vi "Main Process Outgoing Messages.vi"(8 "error in (no error)":errorcluster, 11 "J1939 Main Configuration":T1={"Parameters"={"J1939 XNET Settings"={"XNET Database"="", "XNET Cluster"="", "CAN Port"="", "Baud rate [Bd]"=0, "Termination"=0, "Incoming Rate"=0, "Outcoming Rate"=1, "Write Decimation"=1}, "Incoming Single Point Configuraiton"={"Incoming Single Point Frame"={"ID"=[], "Conversion"=[], "Channel Array Positions"=[], "Frame Length"=[]}, "Channel Pairs"={"Chan Refs"=[], "Previous Chan Values"=[]}, "Read FIFO"=refnum}, "Outgoing Cyclic Configuraiton"={"Outgoing Cyclic Frame"={"ID"=[], "Conversion"=[], "Channel Array Positions"=[], "Frame Length"=[], "Transmit Propreties"=[]}, "Channel Pairs"={"Block Data Refs"=[], "Previous Chan Values"=[]}, "Write FIFO"=refnum}, "J1939 Monitor Settings"={"J1939 Network Address"=0, "Name"=0}, "Simulated Addresses"=[], "Simulated Addresses LUT"=variant, "Name"=""}, "Name"="", "J1939 Cluster"={"Processed Incoming"=refnum, "Current Device Address"=0, "Processed Outgoing"=refnum, "Process Outgoing"=refnum, "Name"=0}, "References"={"BAM Buffer"=refnum, "CM Buffer"=refnum, "CM Gen"=refnum, "BAM Gen"=refnum, "Address Claims"=refnum, "RQST"=refnum}, "Frame In"="", "Frame Out"="", "Incoming Timeout"=0, "Outgoing Timeout"=0, "Listener ID"=refnum, "Process"=refnum, "Data Ref"=refnum, "Scale Ref"=refnum, "Incoming Direct Access"={"Offset"=0, "Length"=0}, "Outgoing Direct Access"={"Offset"=0, "Length"=0}, "TCP Mngr Ref"=refnum, "Name and Address"="", "Simulated Addresses"=[], "Simulated Addresses LUT"=variant} {"Simulated Addresses"."Simulated Addresses"."J1939 XNET Settings"."Name" format="%.0x"; "Simulated Addresses"."Simulated Addresses"."DM1 Data"."Data Reference" format="%.0x"; "Simulated Addresses"."Simulated Addresses"."DM1 Enable?"."Data Reference" format="%.0x"; "Simulated Addresses"."Simulated Addresses"."DM2 Data"."Data Reference" format="%.0x"; "Simulated Addresses"."Simulated Addresses"."DM2 Enable?"."Data Reference" format="%.0x"; "Parameters"."Simulated Addresses"."Simulated Addresses"."J1939 XNET Settings"."Name" format="%.0x"; "Parameters"."J1939 Monitor Settings"."Name" format="%.0x"; "Parameters"."Outgoing Cyclic Configuraiton"."Channel Pairs"."Block Data Refs"."Data Reference" format="%.0x"; "Parameters"."Outgoing Cyclic Configuraiton"."Outgoing Cyclic Frame"."Transmit Propreties"."Transmit Time" format="%#_p"; "Parameters"."J1939 XNET Settings"."Termination" items=["Off", "On"]; "Parameters"."Incoming Single Point Configuraiton"."Channel Pairs"."Chan Refs" format="%.0x"}) -> (0 "error out":errorcluster)   [LabVIEW 2015, in "J1939 Addon Engine.lvlib"]
uses:
  J1939 Addon Engine.lvlib
  Types/Configuration Cluster.ctl
  <vilib>/NI/NI VeriStand Inline Async API/_VS Inline Async API/Process/Process.lvclass
  Types/Process Parameters.ctl
  Shared/Types/XNET Settings.ctl
  Types/Incoming Single Point Configuration.ctl
  Types/Incoming Single Point Frame Pairs.ctl
  Shared/Types/Incoming Single Point Channel Pairs.ctl
  <vilib>/NI Veristand/Custom Device API/Data Reference.ctl
  Types/Outgoing Cyclic Configuration.ctl
  Types/Outgoing Cyclic Frame Pairs.ctl
  Shared/Types/XNET Frame Event Properties.ctl
  Shared/Types/Outgoing Cyclic Channel Pairs.ctl
  <vilib>/NI Veristand/Custom Device API/Block Data Reference.ctl
  Shared/Types/Monitor Settings.ctl
  Types/Simulated Settings.ctl
  Shared/Types/Compiled Simulated Settings.ctl
  Types/DTC FIFOs.ctl
  Shared/J1939 Multi Packet Frame/Types/Setup Information Cluster.ctl
  <vilib>/xnet/xnet.llb/XNET Frame CAN.ctl
  <vilib>/xnet/xnet.llb/XNET Frame Type CAN.ctl
  Shared/J1939 Utilities/Types/CAN Outgoing Message Cluster.ctl
  Shared/J1939 Multi Packet Frame/Types/TP List References.ctl
  Shared/J1939 Multi Packet Frame/Types/BAM Buffer Connections List_Ref.ctl
  Shared/J1939 Multi Packet Frame/Types/TP Buffer Connection Cluster.ctl
  Shared/J1939 Multi Packet Frame/Types/Connection Mode Generation Connection Ref.ctl
  Shared/J1939 Multi Packet Frame/Types/Connection Mode Generation Connection Cluster.ctl
  Shared/J1939 Multi Packet Frame/Types/BAM Generation Connections List_Ref.ctl
  Shared/J1939 Multi Packet Frame/Types/BAM Generation Connection Cluster.ctl
  Shared/J1939 Multi Packet Frame/Types/Address Table Reference.ctl
  Shared/J1939 Multi Packet Frame/Types/RQST Lookup Table Reference.ctl
  Types/Data Lookup Table Reference.ctl
  Types/Datatable Lookup DVR.ctl
  Types/Conversion Lookup Table Reference.ctl
  Shared/J1939 Multi Packet Frame/Types/RQST Comm Lookup Table_Ref.ctl
  Shared/STM/Connection Manager/stm_ManagerStateVariables.ctl
  Shared/STM/TCP/stm_TCP Connection Info.ctl
  Shared/STM/_SubVIs/stm_MetaDataElement.ctl
  Shared/STM/Connection Manager/stm_TCPConnectionProperties.ctl
  Shared/J1939 Multi Packet Frame/J1939 Periodic Messages/SubVIs/Periodic Message Generator Cluster.ctl
  <vilib>/NI/NI VeriStand Inline Async API/_VS Inline Async API/Process/Process.lvclass/Process.ctl
  Shared/J1939 Multi Packet Frame/SubVIs/Read Queued Outgoing Messages.vi
  Shared/J1939 Multi Packet Frame/SubVIs/Process Outgoing Messages by Frame Type.vi
  Shared/J1939 Multi Packet Frame/J1939 Periodic Messages/Periodic Message Generator.vi
  Shared/J1939 Multi Packet Frame/SubVIs/Connection Mode Generation Queue Messages.vi
  <vilib>/NI/NI VeriStand Inline Async API/_VS Inline Async API/Error Handling Process/SubVIs/Error.ConvertArray.vi
  Shared/J1939 Utilities/Check Output Message Frame Type.vi
  Shared/J1939 Multi Packet Frame/J1939 Multi Packet Frames/BAM Generation.vi
  Shared/J1939 Multi Packet Frame/SubVIs/BAM Generation Connections List_Actions.vi
  Shared/J1939 Multi Packet Frame/SubVIs/BAM Generation Create New TP Connection.vi
  Shared/J1939 Multi Packet Frame/J1939 Multi Packet Frames/Connection Mode Generation.vi
  Shared/J1939 Multi Packet Frame/SubVIs/Connection Mode Generation Connections List_Actions.vi
  Shared/J1939 Multi Packet Frame/SubVIs/Connection Mode Generation Search for Connection (Local Message).vi
  Shared/J1939 Multi Packet Frame/SubVIs/Connection Mode Generation Create New TP Connection.vi
  Convert Signals to Frame by ID.vi
  Shared/J1939 Multi Packet Frame/SubVIs/Connection Mode Generation Get Next Messages.vi
  Shared/J1939 Utilities/SubVIs/TP.Conn Abort.vi
  Shared/J1939 Utilities/Common Conversions.vi
  Shared/J1939 Utilities/SubVIs/Convert CAN Arb ID to J1939 ID.vi
  Shared/J1939 Utilities/Common Messages.vi
  Shared/J1939 Utilities/SubVIs/TP.CM BAM.vi
  Shared/J1939 Utilities/SubVIs/TP.DT.vi
  Shared/J1939 Utilities/SubVIs/TP.CM RTS.vi
  Conversion Lookup Table Get Conversion Parameter.vi
  Data Lookup Table Get Signals (Range).vi
  Shared/J1939 Utilities/SubVIs/Convert J1939 ID to CAN Arb ID.vi
  Shared/J1939 Multi Packet Frame/SubVIs/Connection Mode Generation Connections List.vi
  Shared/J1939 Multi Packet Frame/SubVIs/BAM Generation Queue Messages.vi
  Shared/J1939 Multi Packet Frame/SubVIs/BAM Generation Connections List.vi
  Shared/J1939 Multi Packet Frame/SubVIs/BAM Generation Search for Connection (Local Message).vi
  <vilib>/xnet/xnet.llb/XNET Convert.vi
  <vilib>/xnet/xnet.llb/XNET Convert (Signal to Frame Raw).vi
  Data Lookup Table.vi
  Conversion Lookup Table.vi
  Shared/J1939 Utilities/J1939 Utilities.lvlib
  <vilib>/NI VeriStand/Custom Device API/Custom Device API.lvlib
  Shared/J1939 Addon Shared.lvlib
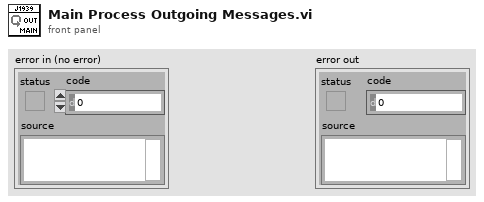
[diagram p1: front panel]
types:
  T1 = typedef "J1939 Addon Engine.lvlib/Configuration Cluster.ctl" = cluster{"Parameters":T2, "Name":string, "J1939 Cluster":T17, "References":T18, "Frame In":refnum<k21>, "Frame Out":refnum<k21>, "Incoming Timeout":u32, "Outgoing Timeout":u32, "Listener ID":refnum<k5>, "Process":refnum<class "Process.lvclass">, "Data Ref":T24, "Scale Ref":T25, "Incoming Direct Access":cluster{"Offset":u32, "Length":u32}, "Outgoing Direct Access":cluster{"Offset":u32, "Length":u32}, "TCP Mngr Ref":T26, "Name and Address":string, "Simulated Addresses":T14[], "Simulated Addresses LUT":variant}
  T2 = typedef "J1939 Addon Engine.lvlib/Process Parameters.ctl" = cluster{"J1939 XNET Settings":T3, "Incoming Single Point Configuraiton":T4, "Outgoing Cyclic Configuraiton":T8, "J1939 Monitor Settings":T13, "Simulated Addresses":T14[], "Simulated Addresses LUT":variant, "Name":string}
  T3 = typedef "J1939 Addon Shared.lvlib/XNET Settings.ctl" = cluster{"XNET Database":refnum<k21>, "XNET Cluster":refnum<k21>, "CAN Port":string, "Baud rate [Bd]":u32, "Termination":u32, "Incoming Rate":u32, "Outcoming Rate":u32, "Write Decimation":u32}
  T4 = typedef "J1939 Addon Engine.lvlib/Incoming Single Point Configuration.ctl" = cluster{"Incoming Single Point Frame":T5, "Channel Pairs":T6, "Read FIFO":refnum<k33>}
  T5 = typedef "J1939 Addon Engine.lvlib/Incoming Single Point Frame Pairs.ctl" = cluster{"ID":u32[], "Conversion":refnum<k21>[], "Channel Array Positions":cluster{"Offset":u32, "Length":u32}[], "Frame Length":u32[]}
  T6 = typedef "J1939 Addon Shared.lvlib/Incoming Single Point Channel Pairs.ctl" = cluster{"Chan Refs":T7[], "Previous Chan Values":dbl[]}
  T7 = typedef "Custom Device API.lvlib/Data Reference.ctl" = i32
  T8 = typedef "J1939 Addon Engine.lvlib/Outgoing Cyclic Configuration.ctl" = cluster{"Outgoing Cyclic Frame":T9, "Channel Pairs":T11, "Write FIFO":refnum<k33>}
  T9 = typedef "J1939 Addon Engine.lvlib/Outgoing Cyclic Frame Pairs.ctl" = cluster{"ID":u32[], "Conversion":refnum<k21>[], "Channel Array Positions":cluster{"Offset":u32, "Length":u32}[], "Frame Length":u32[], "Transmit Propreties":T10[]}
  T10 = typedef "J1939 Addon Shared.lvlib/XNET Frame Event Properties.ctl" = cluster{"Transmit trigger":enum16{"Channel value change"}, "Enable software cyclic trigger":bool, "Transmit Time":dbl}
  T11 = typedef "J1939 Addon Shared.lvlib/Outgoing Cyclic Channel Pairs.ctl" = cluster{"Block Data Refs":T12[], "Previous Chan Values":dbl[]}
  T12 = typedef "Custom Device API.lvlib/Block Data Reference.ctl" = cluster{"Data Reference":T7, "Offset":u64, "Length":u64}
  T13 = typedef "J1939 Addon Shared.lvlib/Monitor Settings.ctl" = cluster{"J1939 Network Address":u8, "Name":u64}
  T14 = typedef "J1939 Addon Engine.lvlib/Simulated Settings.ctl" = cluster{"Simulated Addresses":T15, "FIFOs":T16}
  T15 = typedef "J1939 Addon Shared.lvlib/Compiled Simulated Settings.ctl" = cluster{"J1939 XNET Settings":T13, "DM1 Data":T12[], "DM1 Data":dbl[], "DM1 Enable?":T12[], "DM1 Enable?":dbl[], "DM2 Data":T12[], "DM2 Data":dbl[], "DM2 Enable?":T12[], "DM2 Enable?":dbl[]}
  T16 = typedef "J1939 Addon Engine.lvlib/DTC FIFOs.ctl" = cluster{"DM1 Data":refnum<k33>, "DM1 Enable?":refnum<k33>, "DM2 Data":refnum<k33>, "DM2 Enable?":refnum<k33>, "DM1 Reset?":refnum<k33>, "DM2 Reset?":refnum<k33>}
  T17 = typedef "J1939 Addon Engine.lvlib/Setup Information Cluster.ctl" = cluster{"Processed Incoming":refnum<queue>, "Current Device Address":u8, "Processed Outgoing":refnum<queue>, "Process Outgoing":refnum<queue>, "Name":u64}
  T18 = typedef "J1939 Addon Engine.lvlib/TP List References.ctl" = cluster{"BAM Buffer":T19, "CM Buffer":T19, "CM Gen":T20, "BAM Gen":T21, "Address Claims":T22, "RQST":T23}
  T19 = typedef "J1939 Addon Engine.lvlib/BAM Buffer Connections List_Ref.ctl" = refnum<data-value>
  T20 = typedef "J1939 Addon Engine.lvlib/Connection Mode Generation Connection Ref.ctl" = refnum<data-value>
  T21 = typedef "J1939 Addon Engine.lvlib/BAM Generation Connections List_Ref.ctl" = refnum<data-value>
  T22 = typedef "J1939 Addon Engine.lvlib/Address Table Reference.ctl" = refnum<data-value>
  T23 = typedef "J1939 Addon Engine.lvlib/RQST Lookup Table Reference.ctl" = refnum<data-value>
  T24 = typedef "J1939 Addon Engine.lvlib/Data Lookup Table Reference.ctl" = refnum<data-value>
  T25 = typedef "J1939 Addon Engine.lvlib/Conversion Lookup Table Reference.ctl" = refnum<data-value>
  T26 = typedef "J1939 Addon Shared.lvlib/RQST Comm Lookup Table_Ref.ctl" = refnum<data-value>
  T27 = typedef "J1939 Addon Engine.lvlib/Periodic Message Generator Cluster.ctl" = cluster{"Arb ID":u32, "Timeout":u32, "Start Timeout":u32}
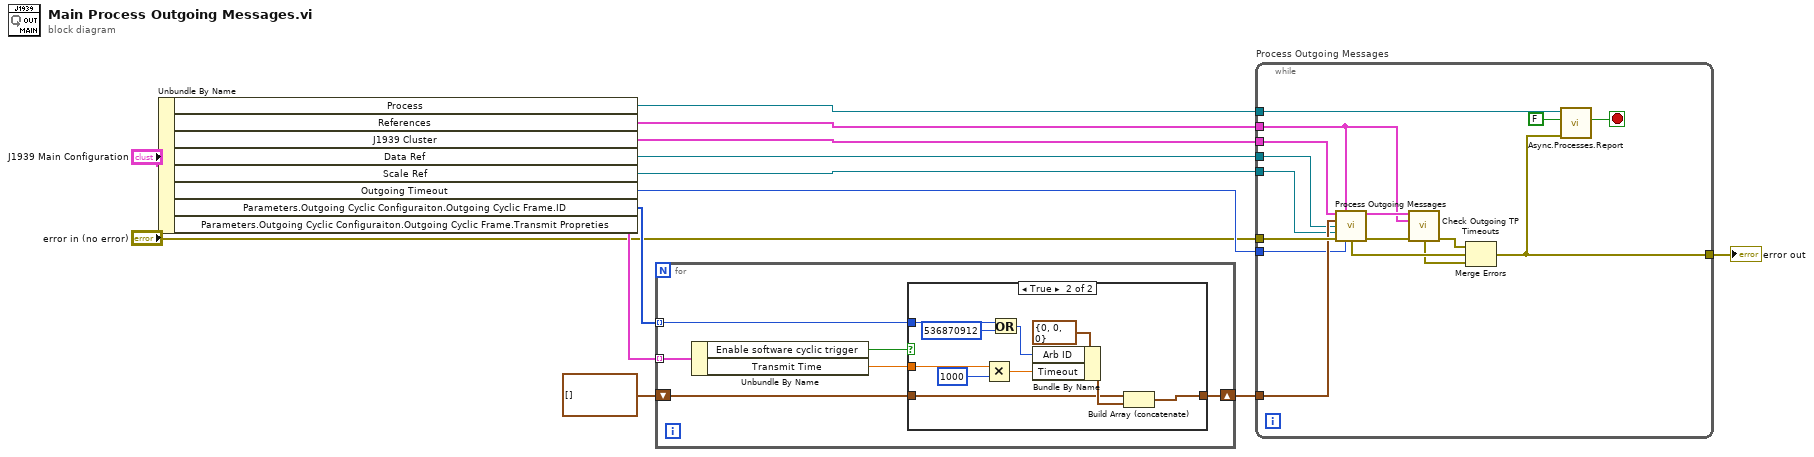
[diagram p0: block diagram]
diagram:
  n1 = Unbundle By Name("J1939 Main Configuration") -> ("Process"=w5:refnum<class "Process.lvclass">, "References"=w6:T18, "J1939 Cluster"=w7:T17, "Data Ref"=w8:T24, "Scale Ref"=w9:T25, "Outgoing Timeout"=w4:u32, "Parameters.Outgoing Cyclic Configuraiton.Outgoing Cyclic Frame.ID"=w12:u32[], "Parameters.Outgoing Cyclic Configuraiton.Outgoing Cyclic Frame.Transmit Propreties"=w11:T10[])
  n2 = for {
    tunnel: w12 -> [w19] mode=indexing
    tunnel: w11 -> [w17] mode=indexing
    shift-right: [w18] -> w13
    shift-left: T27[] [] -> [w14]
    n3 = Unbundle By Name(w17) -> ("Enable software cyclic trigger"=w16:bool, "Transmit Time"=w15:dbl)
    n4 = case shown="True" w16 {
      tunnel: w19 -> [_ w22]
      tunnel: [w20 w25] -> w18
      tunnel: w15 -> [_ w27]
      tunnel: w14 -> [w20 w24]
      frame False {
      }
      frame True {
        n5 = Multiply(x=w27, y=1000) -> (x*y=w26:dbl)
        n6 = Or(x=w22, y=u32 536870912) -> (x .or. y?=w21:u32)
        n7 = Bundle By Name(cluster=T27 {"Arb ID"=0, "Timeout"=0, "Start Timeout"=0}, "Arb ID"=w21, "Timeout"=w26) -> (w29:T27)
        n8 = Build Array (concatenate)(w24, w29) -> (w25:T27[])
      }
    }
  }
  n9 = while "Process Outgoing Messages" {
    tunnel: w7 -> [w44]
    tunnel: [w31] -> w1
    tunnel: "error in (no error)" -> [w43]
    tunnel: w13 -> [w41]
    tunnel: w8 -> [w38]
    tunnel: w9 -> [w39]
    tunnel: w6 -> [w37]
    tunnel: w4 -> [w33]
    tunnel: w5 -> [w32]
    stop <- w42 stop-if-true
    n10 = call "Process Outgoing Messages.vi"("J1939 Cluster"=w44, "Connection Refs"=w37, "Timeouts"=w41, "Data Ref"=w38, "Scale Ref"=w39, "error in"=w43, "timeout in ms (-1)"=w33) -> ("J1939 Cluster Out"=w45:T17, "Message Errors"=w36:errorcluster, "error out"=w46:errorcluster)  [unwired: 6 out]
    n11 = call "Check Outgoing TP Timeouts.vi"("J1939 Cluster"=w45, "Connection Refs"=w37, "error in"=w46) -> ("Message Error"=w35:errorcluster, "error out"=w34:errorcluster)  [unwired: 11 out]
    n12 = Merge Errors(w34, w36, w35) -> (w31:errorcluster)
    n13 = call <vilib>:"Async.Processes.Report.vi"("Error"=w31, "Stop on Error?"=FALSE, "Process in"=w32) -> ("Stop"=w42:bool)  [unwired: 7 in, 1 out]
  }
  "error out" <- w1
